vi "solar_excel File Write (Sheet).vi"(6 "Visible? (F)":bool, 7 "Worksheet":string, 8 "error in (no error)":errorcluster, 9 "Cells":string[][](array[string]), 10 "Start (1,1 = 'A1')":cluster{"Row":u32, "Column":u32}, 11 "Excel Workbook (*.xlsx)":path) -> (0 "error out":errorcluster, 3 "dup Excel Workbook":path)   [LabVIEW 2018]
doc: "This appends a cell range to an Excel Workbook (*.xlsx) specified by the <b>Start</b> cell range and size of the <b>Cells</b> to append."
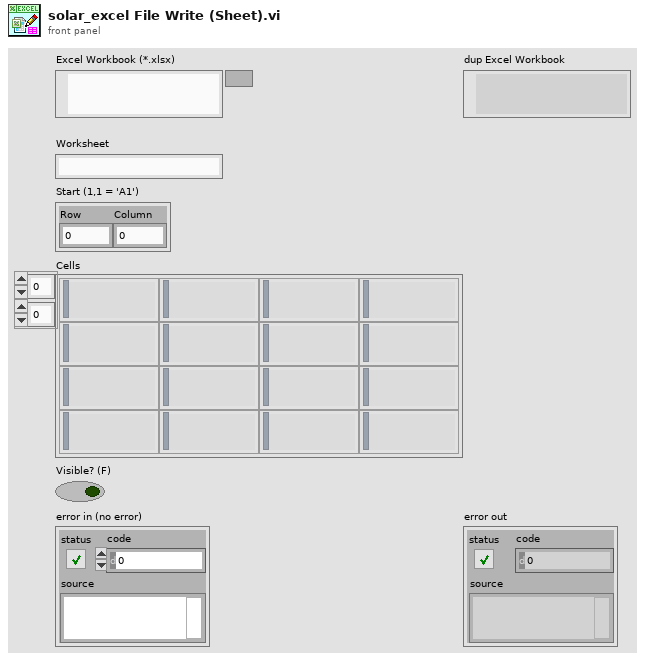
[diagram p1: front panel]
types:
  T1 = typedef "solar_excel_ctl App.ctl" = cluster{"ExcelApp":refnum<k7>, "Workbooks":refnum<k7>, "TSV":refnum<queue>}
  T2 = typedef "solar_excel_ctl Workbook.ctl" = cluster{"ExcelApp":refnum<k7>, "Workbooks":refnum<k7>, "TSV":refnum<queue>, "OpenWkb":refnum<k7>}
  T3 = typedef "solar_excel_ctl Worksheet.ctl" = cluster{"ExcelApp":refnum<k7>, "Workbooks":refnum<k7>, "TSV":refnum<queue>, "OpenWkb":refnum<k7>, "Worksheets":refnum<k7>, "OpenWksh":refnum<k7>}
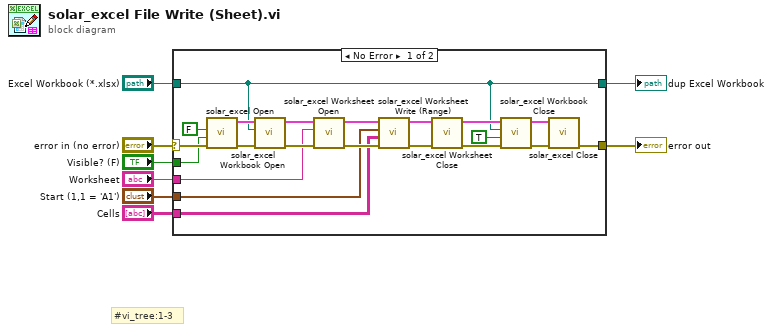
[diagram p0: block diagram]
diagram:
  # "#vi_tree:1-3"
  n1 = case shown="No Error" "error in (no error)" {
    selector: "error in (no error)" -> [w22 w31]
    tunnel: [w23 w31] -> w8
    tunnel: "Visible? (F)" -> [w21 _]
    tunnel: "Excel Workbook (*.xlsx)" -> [w15 w30]
    tunnel: "Worksheet" -> [w16 _]
    tunnel: [w15 w30] -> w3
    tunnel: "Start (1,1 = 'A1')" -> [w10 _]
    tunnel: "Cells" -> [w9 _]
    frame No Error {
      n2 = call "solar_excel Open.vi"("error in (no error)"=w22, "Visible? (F)"=w21, "Open New Instance? (F)"=FALSE) -> ("error out"=w28:errorcluster, "Excel App"=w29:T1)  [unwired: 7 in]
      n3 = call "solar_excel Workbook Open.vi"("error in (no error)"=w28, "Excel Workbook (*.xlsx)"=w15, "Excel App"=w29) -> ("error out"=w17:errorcluster, "Excel Workbook"=w18:T2)  [unwired: 7 in]
      n4 = call "solar_excel Worksheet Open.vi"("error in (no error)"=w17, "Sheet Name (STR) or Number (I32)"=w16, "Excel Workbook"=w18) -> ("error out"=w13:errorcluster, "Excel Worksheet"=w14:T3)  [unwired: 5 in, 2 out]
      n5 = call "solar_excel Worksheet Write (Range).vi"("error in (no error)"=w13, "Cells"=w9, "Start (1,1 = 'A1')"=w10, "Excel Worksheet in"=w14) -> ("error out"=w12:errorcluster, "Excel Worksheet out"=w11:T3)  [unwired: 6 in]
      n6 = call "solar_excel Worksheet Close.vi"("error in (no error)"=w12, "Excel Worksheet"=w11) -> ("error out"=w27:errorcluster, "Excel Workbook"=w26:T2)  [unwired: 8 in]
      n7 = call "solar_excel Workbook Close.vi"("error in (no error)"=w27, "Save? (F)"=TRUE, "Excel Workbook (*.xlsx)"=w15, "Excel Workbook"=w26) -> ("error out"=w25:errorcluster, "Excel App"=w24:T1)  [unwired: 6 in]
      n8 = call "solar_excel Close.vi"("error in (no error)"=w25, "Excel App"=w24) -> ("error out"=w23:errorcluster)  [unwired: 9 in]
    }
    frame Error {
    }
  }
  "error out" <- w8
  "dup Excel Workbook" <- w3
